vi "Destructor.vi"(8 "error in":errorcluster, 11 "ProductUnit in":refnum<class "ProductUnit.lvclass">) -> (0 "error out":errorcluster)   [LabVIEW 2021, in "ProligentXMLGenerator.lvlib" / "ProductUnit.lvclass"]
uses:
  ProductUnit.lvclass
  ProductUnit.lvclass/ProductUnit.ctl
  Model/CustomData/CustomData.lvclass
  Model/Characteristic/Characteristic.lvclass
  Model/Document/Document.lvclass
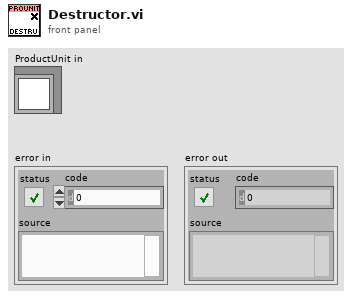
[diagram p1: front panel]
types:
  T1 = typedef "ProligentXMLGenerator.lvlib/ProductUnit.lvclass/Data.ctl" = cluster{"Name":string, "Characteristics":refnum<class "Characteristic.lvclass">[], "Documents":refnum<class "Document.lvclass">[], "CustomData":refnum<class "CustomData.lvclass">, "ProductUnitIdentifier":refnum<class "NonEmptyString_50.lvclass">, "ProductFullName":refnum<class "FullName.lvclass">, "Scrapped":refnum<class "Boolean.lvclass">, "ScrappedTime":refnum<class "DateTime.lvclass">, "CreationTime":refnum<class "DateTime.lvclass">, "ManufacturingTime":refnum<class "DateTime.lvclass">, "ByManufacturer":refnum<class "NonEmptyString_255.lvclass">, "TimeZoneInfoId":string}
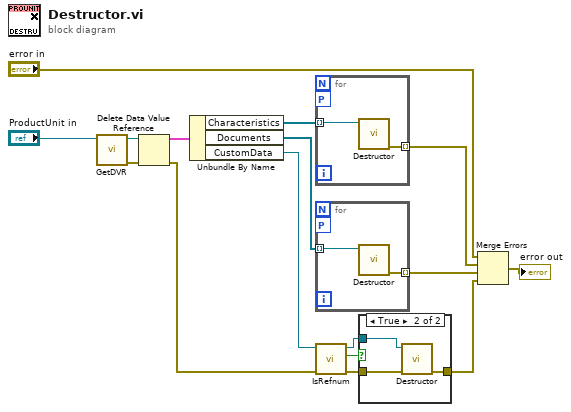
[diagram p0: block diagram]
diagram:
  n1 = call "GetDVR.vi"("ProductUnit in"="ProductUnit in") -> ("error out"=w13:errorcluster, "DVRReference"=w14:refnum<data-value>)  [unwired: 9 in]
  n2 = Delete Data Value Reference(data value reference=w14, error in=w13) -> (data value=w12:T1, error out=w1:errorcluster)
  n3 = Unbundle By Name(w12) -> ("Characteristics"=w9:refnum<class "Characteristic.lvclass">[], "Documents"=w8:refnum<class "Document.lvclass">[], "CustomData"=w3:refnum<class "CustomData.lvclass">)
  n4 = for {
    tunnel: w9 -> [w18] mode=indexing
    tunnel: [w17] -> w10 mode=indexing
    workers-P: _ -> [_]
    n5 = call "Destructor.vi"("Document in"=w18) -> ("error out"=w17:errorcluster)  [unwired: 10 in]
  }
  n6 = for {
    tunnel: w8 -> [w20] mode=indexing
    tunnel: [w19] -> w7 mode=indexing
    workers-P: _ -> [_]
    n7 = call "Destructor.vi"("Document in"=w20) -> ("error out"=w19:errorcluster)  [unwired: 10 in]
  }
  n8 = call "IsRefnum.vi"("error in"=w1, "CustomDataType in"=w3) -> ("error out"=w4:errorcluster, "IsRefnum"=w6:bool, "CustomDataType out"=w5:refnum<class "CustomData.lvclass">)  [unwired: 7 in]
  n9 = case shown="True" w6 {
    tunnel: w5 -> [_ w24]
    tunnel: w4 -> [w21 w23]
    tunnel: [w21 w22] -> w2
    frame False {
    }
    frame True {
      n10 = call "Destructor.vi"("error in"=w23, "CustomDataType"=w24) -> ("error out"=w22:errorcluster)  [unwired: 9 in]
    }
  }
  n11 = Merge Errors("error in", w10, w7, w2) -> (→"error out":errorcluster)
